vi "读取系列号.vi"(8 "Error in":errorcluster caption="Error in (no error)", 11 "站号":u16(ring)=10 items=["氨氮"=3, "水温"=9, "pH值"=10, "溶解氧"=11, "电导率"=12, "浊度"=13, "叶绿素a"=14, "藻密度"=15, "蓝绿藻"=16, "氧化还原电位"=17, "溶解氧%"=18, "盐度"=19]) -> (0 "error out":errorcluster, 3 "SN":string)   [LabVIEW 2016, in "斯坦道原位多参数.lvlib"]
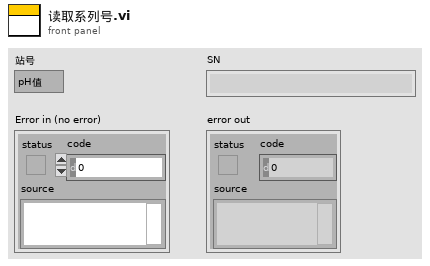
[diagram p1: front panel]
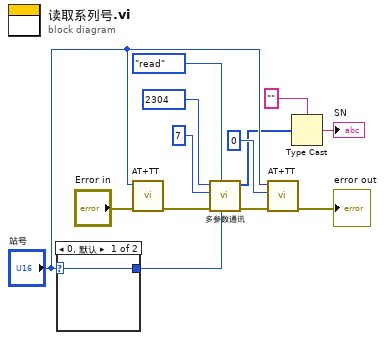
[diagram p0: block diagram]
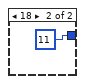
[diagram p2: hidden frame]
diagram:
  n1 = case shown="0, 默认" "站号" {
    selector: "站号" -> [w14 _]
    tunnel: [w14 u16 11 ("站号")] -> w8
    frame 0, Default {
    }
    frame 18 {
    }
  }
  n2 = call "AT+TT.vi"("错误输入（无错误）"="Error in", "站号"="站号") -> ("错误输出"=w9:errorcluster)  [unwired: 9 in]
  n3 = call "多参数通讯.vi"("Slave ID"=w8, "STEP"=enum16{"open", "read", "write", "close"}."read", "Error in"=w9, "quantity"=u16 7, "starting address"=u16 2304) -> ("error out"=w7:errorcluster, "Registers"=w2:u16[])  [unwired: 4 in, 1 out]
  n4 = call "AT+TT.vi"("错误输入（无错误）"=w7, "Count"=0, "站号"="站号") -> ("错误输出"=→"error out":errorcluster)  [unwired: 8 in]
  n5 = Type Cast(type="", x=w2) -> (*(type *) &x=→"SN":string)
